vi "Serialize Args for Windows.vi"(8 "error in":errorcluster, 11 "Args":string[](array[string])) -> (0 "error out":errorcluster, 3 "String":string)   [LabVIEW 2025, in "Process Executor.lvclass"]
doc: "Converts an array of tokenized command-line arguments into a single Windows-compatible argument string.\n\nThe VI applies quoting and escaping rules to each argument as needed, ensuring correct handling of spaces, quotes, and backslashes, and then concatenates the serialized tokens in the proper order."
uses:
  Process Executor.lvclass
  Process Executor.lvclass/Process Executor.ctl
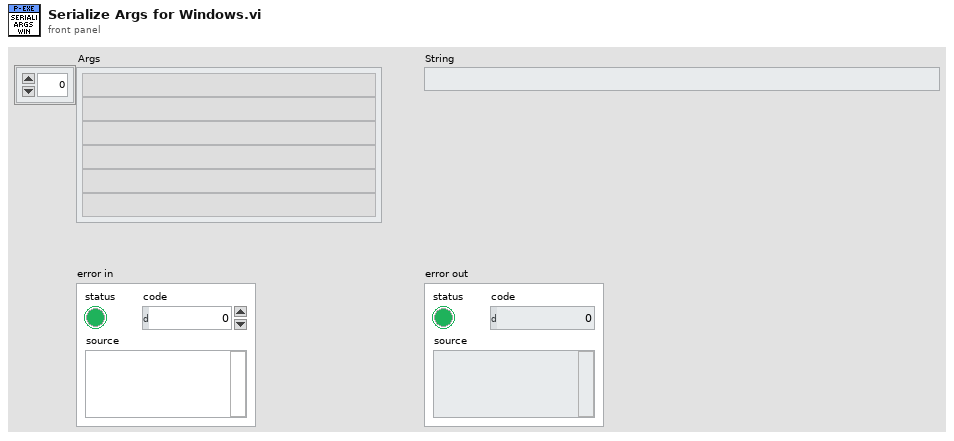
[diagram p1: front panel]
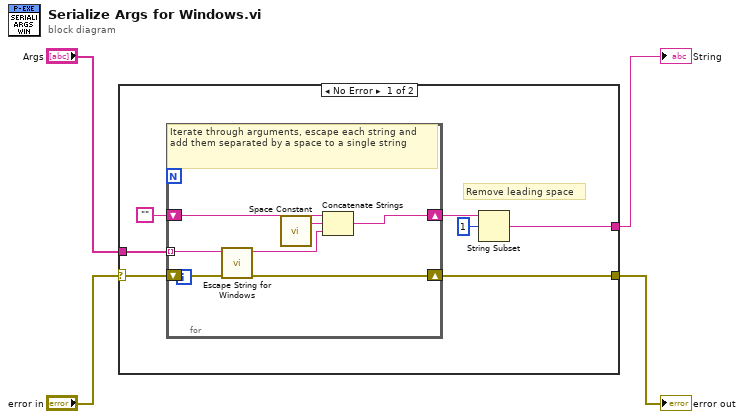
[diagram p0: block diagram]
diagram:
  n1 = case shown="No Error" "error in" {
    selector: "error in" -> [w11 w19]
    tunnel: "Args" -> [w8 _]
    tunnel: [w10 w19] -> w3
    tunnel: [w5 _] -> w1
    frame No Error {
      # "Remove leading space"
      n2 = for {
        tunnel: w8 -> [w14] mode=indexing
        shift-right: [w15] -> w7
        shift-left: "" ("Empty String Constant") -> [w16]
        shift-right: [w17] -> w10
        shift-left: w11 -> [w18]
        # "Iterate through arguments, escape each string and add them separated by a space to a single string"
        n3 = call "Escape String for Windows.vi"("error in"=w18, "String in"=w14) -> ("error out"=w17:errorcluster, "String out"=w13:string)  [unwired: 8 in]
        n4 = call <vilib>:"Space Constant.vi"() -> ("String"=w12:string)
        n5 = Concatenate Strings(w16, w12, w13) -> (w15:string)
      }
      n6 = String Subset(string=w7, offset (0)=1) -> (substring=w5:string)  [unwired: 1 in]
    }
    frame Error {
      # "Pass error without further action"
    }
  }
  "error out" <- w3
  "String" <- w1
